vi "ex7-7.vi"() -> ()   [LabVIEW 2013]
panel:
  out "output array":dbl[](array[numeric])
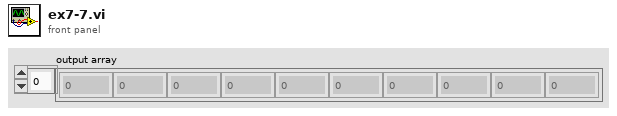
[diagram p1: front panel]
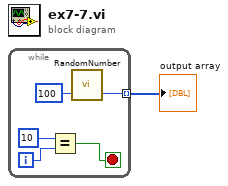
[diagram p0: block diagram]
diagram:
  n1 = while {
    tunnel: [w6] -> w1 mode=indexing
    i -> [w4]
    stop <- w2 stop-if-true
    n2 = Equal?(x=10, y=w4) -> (x = y?=w2:bool)
    n3 = call <vilib>:"RandomNumber.vi"("Max Value"=u16 100) -> ("Random Number"=w6:u16)  [unwired: 2 in, 1 out]
  }
  "output array" <- w1
